vi "USB RAW - Interrupt.vi"() -> ()   [LabVIEW 2023]
doc: "This example shows how to use interrupts with a USB RAW device. \n\n<b>Note:</b> This example works only with USB RAW devices.\n\nBefore you run this VI, install a USB RAW device and configure NI Measurement & Automation Explorer (MAX) to recognize the USB device. You can enable and wait for an interrupt on a USB RAW device only after you install and configure the USB RAW device and open a session to the device.\n\nTo use another device, close the session to the current device, select another device from the <b>VISA Resource</b> control, and open a session to the new device. \n\nWhen the interrupt is complete, click the <b>Stop</b> button to stop the VI."
uses:
  <vilib>/Instr/_visa.llb/Select Event Type.ctl
panel:
  in  "Not USB":string="The specified VISA resource is not a USB device."
  in  "Timeout (ms)":u32=10000
  out "Interrupt Data":u8[](array[numeric]) format="%.0x"
  in  "Stop":bool
  in  "VISA Resource":refnum<visa-resource-name>
  in  "Enable and Wait for Interrupt":bool
  # "Overview: Demonstrates the use of the VISA Get USB Interrupt Data VI to retrieve interrupt data from a USB RAW device.\nRequirements: NI-VISA Driver, USB RAW device\nInstructions:\n1. Ensure the USB RAW device specified by the VISA Resource control is properly configured in Measurement & Automation Explorer. For the type of interrupt pipe device required for this example, that may require additional operating system configuration of the device, as well as the use of the VISA Driver Development Wizard.\n2. Run the VI.\n3. Click Enable and Wait for Interrupt, and view the Interrupt Data returned by the device.\n4. Click Stop to stop the VI."
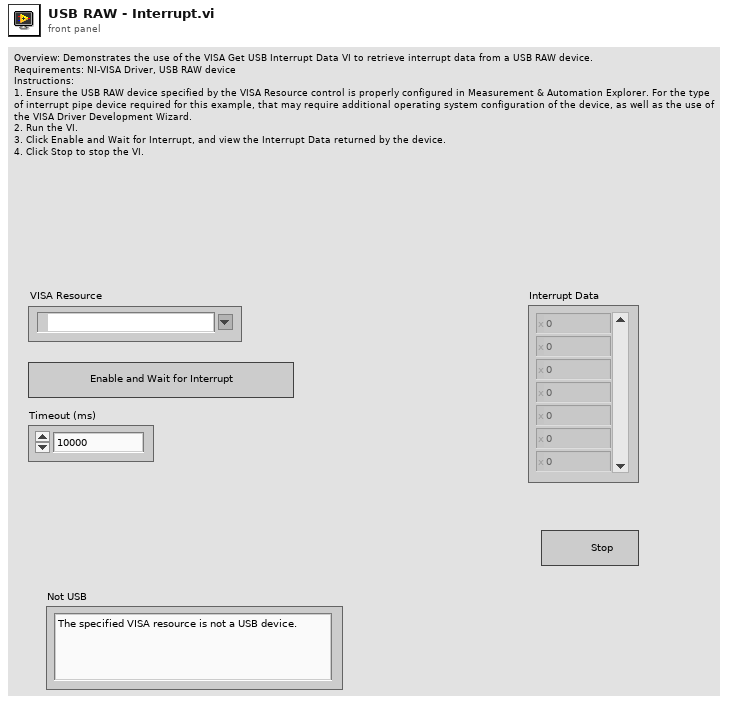
[diagram p1: front panel]
types:
  T1 = typedef "Select Event Type.ctl" = u32
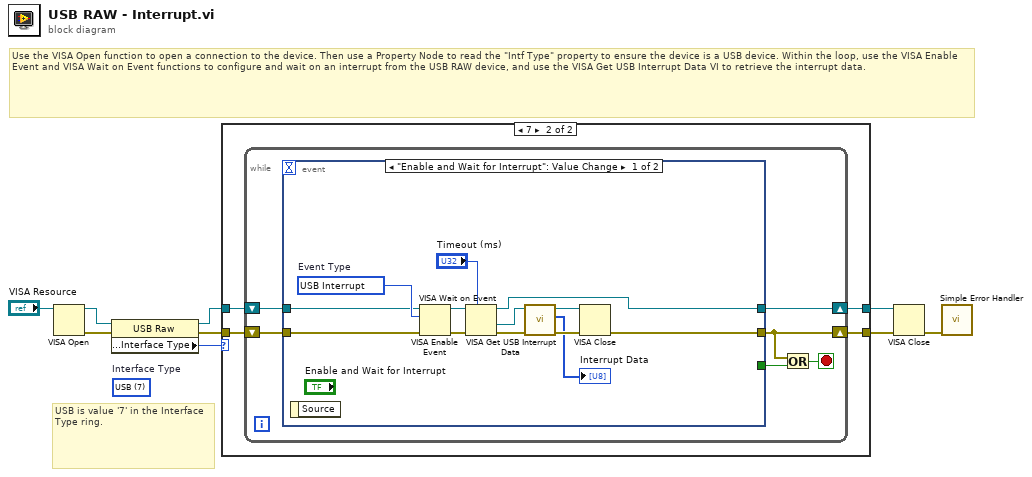
[diagram p0: block diagram]
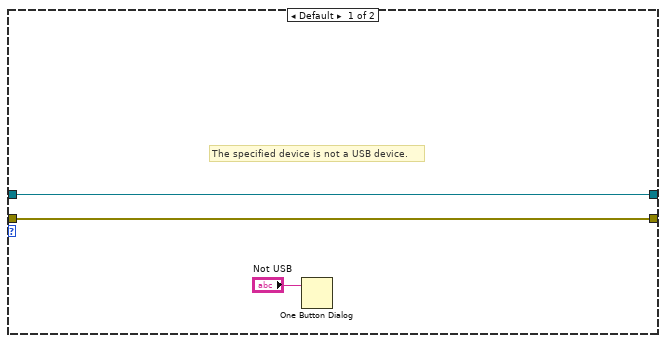
[diagram p2: hidden frame]
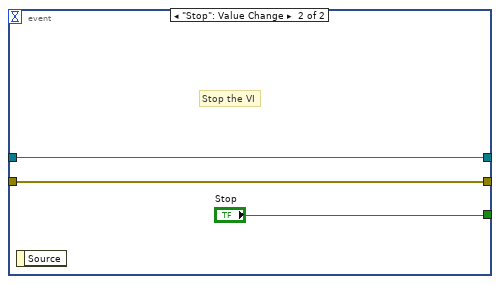
[diagram p3: hidden frame]
diagram:
  (unwired) u16 7 items=["GPIB"=1, "VXI"=2, "GPIB-VXI"=3, "Serial"=4, "PXI"=5, "TCPIP"=6, "USB"=7, "FireWire"=9]  # Interface Type
  # "Use the VISA Open function to open a connection to the device. Then use a Property Node to read the \"Intf Type\" property to ensure the device is a USB device. Within the loop, use the VISA Enable Event and VISA Wait on Event functions to configure and wait on an interrupt from the USB RAW device, and use the VISA Get USB Interrupt Data VI to retrieve the interrupt data."
  # "USB is value '7' in the Interface Type ring."
  n1 = VISA Open(VISA resource name="VISA Resource") -> (VISA resource name=w3:refnum<visa-resource-name>, error out=w6:errorcluster)  [unwired: 1 in, 3 out]
  n2 = property class="USB Raw"(reference=w3, error in=w6) -> (reference out=w4:refnum<visa-resource-name>, error out=w5:errorcluster, "Interface Information:Interface Type"=w1:u16)
  n3 = case shown="7" w1 {
    tunnel: [w12 w16] -> w9
    tunnel: [w11 w15] -> w7
    tunnel: w5 -> [w12 w14]
    tunnel: w4 -> [w11 w13]
    frame Default {
      # "The specified device is not a USB device."
      n4 = One Button Dialog(message="Not USB") -> ()  [unwired: 1 in, 1 out]
    }
    frame 7 {
      n5 = while {
        shift-right: [w18] -> w16
        shift-left: w14 -> [w17]
        shift-right: [w20] -> w15
        shift-left: w13 -> [w19]
        stop <- w21 stop-if-true
        n6 = event shown="[0] \"Enable and Wait for Interrupt\": Value Change" {
          selector: _ -> [_ _]
          dyn-events: _ -> [_ _]
          timeout: _ -> [_ _]
          tunnel: [_ "Stop"] -> w22
          tunnel: [w25 w37] -> w18
          tunnel: w17 -> [w26 w37]
          tunnel: [w23 w36] -> w20
          tunnel: w19 -> [w27 w36]
          event "Enable and Wait for Interrupt": Value Change {
            w28 = T1 1073684535 items=["Service Request"=1073684491, "Trigger"=3221168138, "Clear"=1073684493, "VXI Signal"=1073684512, "VXI/VME Interrupt"=3221168161, "VXI/VME Sysfail"=1073684509, "VXI/VME Sysreset"=1073684510, "GPIB CIC"=1073684498, "GPIB Talk"=1073684499, "GPIB Listen"=1073684500, "PXI Interrupt"=1073684514, "Serial Break"=1073684515, "Serial TermChar"=1073684516, "Serial CTS"=1073684521, "Serial DSR"=1073684522, "Serial DCD"=1073684524, "Serial RI"=1073684526, "Serial Character"=1073684533, "USB Interrupt"=1073684535, "All Enabled"=1073709055]  # Event Type
            n7 = event-data() -> ()  [unwired: 2 out]
            n8 = VISA Enable Event(8:w26, 10:w28, 11:w27) -> (0:w34:errorcluster, 3:w35:refnum<visa-resource-name>)  [unwired: 1 out]
            n9 = VISA Wait on Event(7:"Timeout (ms)", 8:w34, 11:w35) -> (0:w32:errorcluster, 1:w33:refnum<visa-resource-name>, 3:w23:refnum<visa-resource-name>)  [unwired: 3 out]
            n10 = call <vilib>:"VISA Get USB Interrupt Data.vi"("error in (no error)"=w32, "VISA USB Intr Event"=w33) -> ("error out"=w31:errorcluster, "data buffer"=→"Interrupt Data":u8[], "VISA USB Intr Event out"=w30:refnum<visa-resource-name>)  [unwired: 7 out]
            n11 = VISA Close(VISA resource name=w30, error in (no error)=w31) -> (error out=w25:errorcluster)
          }
          event "Stop": Value Change {
            # "Stop the VI"
            n12 = event-data() -> ()  [unwired: 2 out]
          }
        }
        n13 = Or(x=w18, y=w22) -> (x .or. y?=w21:bool)
      }
    }
  }
  n14 = VISA Close(VISA resource name=w7, error in (no error)=w9) -> (error out=w8:errorcluster)
  n15 = call <vilib>:"Simple Error Handler.vi"("error in (no error)"=w8) -> ()  [unwired: 1 in, 8 out]
